vi "Test MQTT-2.2.2-1.vi"(8 "error in (no error)":errorcluster) -> (0 "error out":errorcluster)   [LabVIEW 2013]
uses:
  <vilib>/LabVIEW Open Source Project/MQTT Control Packets/Control Packets/CONNECT/ConnectFlags -- cluster.ctl
  <vilib>/LabVIEW Open Source Project/MQTT Control Packets/Control Packets/SUBACK/Subscription Success Code.ctl
  <vilib>/LabVIEW Open Source Project/MQTT Control Packets/Control Packets/ControlPacket/QualityOfService -- enum.ctl
  <vilib>/LabVIEW Open Source Project/MQTT Control Packets/Control Packets/SUBSCRIBE/Topic Subscription -- cluster.ctl
  <vilib>/LabVIEW Open Source Project/MQTT Control Packets/Control Packets/ControlPacket/ControlPacket.lvclass/ControlPacket.ctl
  <vilib>/addons/_JKI Toolkits/Caraya/classes/Assert/Assert True.vi
  <vilib>/addons/_JKI Toolkits/Caraya/classes/Test/Test.lvclass
  <vilib>/LabVIEW Open Source Project/MQTT Control Packets/Control Packets/ControlPacket/ControlPacket.lvclass
  <vilib>/addons/_JKI Toolkits/Caraya/classes/Assert/Assert.lvclass
  <vilib>/LabVIEW Open Source Project/MQTT Control Packets/Control Packets/CONNECT/CONNECT.lvclass
  <vilib>/LabVIEW Open Source Project/MQTT Control Packets/Control Packets/CONNACK/CONNACK.lvclass
  <vilib>/LabVIEW Open Source Project/MQTT Control Packets/Control Packets/DISCONNECT/DISCONNECT.lvclass
  <vilib>/LabVIEW Open Source Project/MQTT Control Packets/Control Packets/PINGREQ/PINGREQ.lvclass
  <vilib>/LabVIEW Open Source Project/MQTT Control Packets/Control Packets/PINGRESP/PINGRESP.lvclass
  <vilib>/LabVIEW Open Source Project/MQTT Control Packets/Control Packets/PUBACK/PUBACK.lvclass
  <vilib>/LabVIEW Open Source Project/MQTT Control Packets/Control Packets/PUBCOMP/PUBCOMP.lvclass
  <vilib>/LabVIEW Open Source Project/MQTT Control Packets/Control Packets/UNSUBSCRIBE/UNSUBSCRIBE.lvclass
  <vilib>/LabVIEW Open Source Project/MQTT Control Packets/Control Packets/UNSUBACK/UNSUBACK.lvclass
  <vilib>/LabVIEW Open Source Project/MQTT Control Packets/Control Packets/SUBSCRIBE/SUBSCRIBE.lvclass
  <vilib>/LabVIEW Open Source Project/MQTT Control Packets/Control Packets/SUBACK/SUBACK.lvclass
  <vilib>/LabVIEW Open Source Project/MQTT Control Packets/Control Packets/PUBREL/PUBREL.lvclass
  <vilib>/LabVIEW Open Source Project/MQTT Control Packets/Control Packets/PUBREC/PUBREC.lvclass
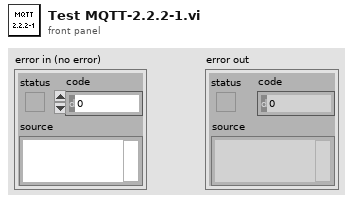
[diagram p1: front panel]
types:
  T1 = typedef "MQTT_Control_Packets.lvlib/SUBSCRIBE.lvclass/Topic Subscription -- cluster.ctl" = cluster{"Topic Filter":string, "QoS":T2}
  T2 = typedef "MQTT_Control_Packets.lvlib/ControlPacket.lvclass/QualityOfService -- enum.ctl" = enum16{"0 (At Most Once)", "1 (At Least Once)", "2 (Exactly Once)"}
  T3 = typedef "MQTT_Control_Packets.lvlib/SUBACK.lvclass/Subscription Success Code.ctl" = cluster{"Subscription Failure":bool, "QoS":T2}
  T4 = typedef "MQTT_Control_Packets.lvlib/CONNECT.lvclass/ConnectFlags -- cluster.ctl" = cluster{"Reserved":bool, "Clean Session":bool, "Will Flag":bool, "Will QoS 1":bool, "Will QoS 2":bool, "Will Retain":bool, "Password Flag":bool, "User Name Flag":bool}
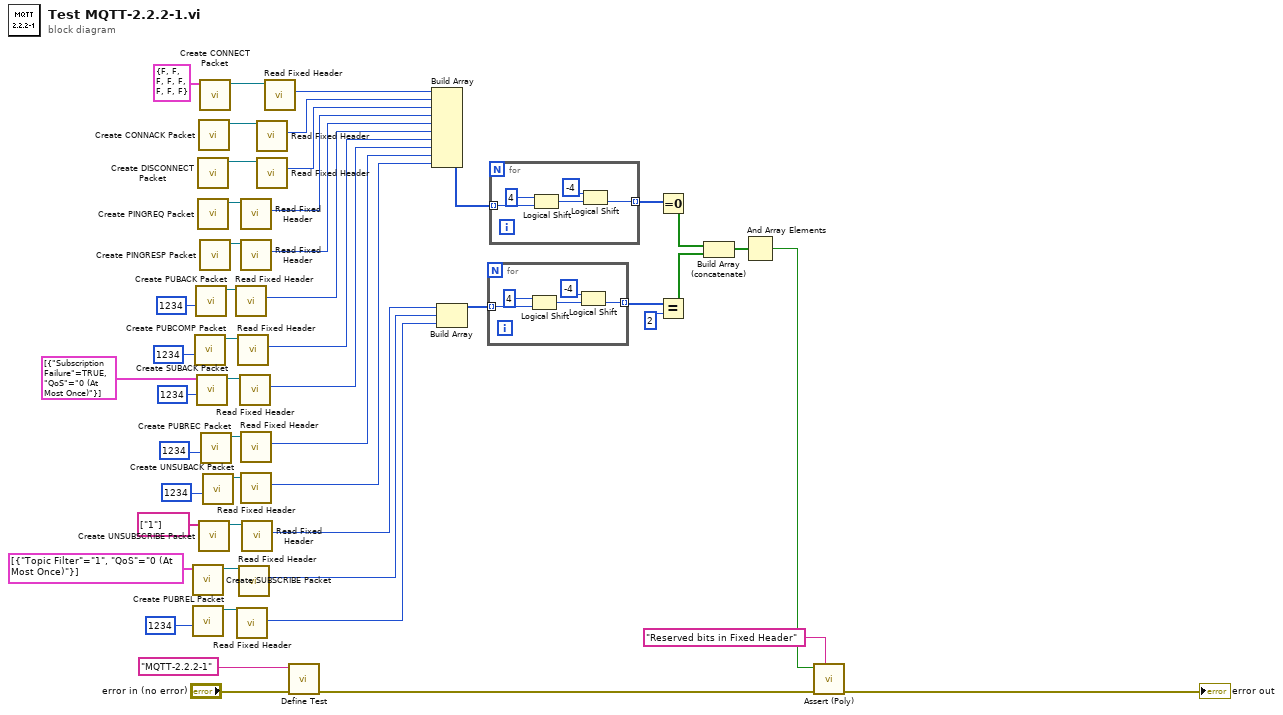
[diagram p0: block diagram]
diagram:
  n1 = call <vilib>:"Create SUBSCRIBE Packet.vi"("Topic Subscriptions"=T1[] [{"Topic Filter"="1", "QoS"=enum."0 (At Most Once)"}]) -> ("SUBSCRIBE out"=w24:refnum<class "SUBSCRIBE.lvclass">)  [unwired: 9 in, 1 out]
  n2 = call <vilib>:"Create PUBREL Packet.vi"("Packet ID"=u16 1234) -> ("PUBREL out"=w31:refnum<class "PUBREL.lvclass">)  [unwired: 9 in, 1 out]
  n3 = call <vilib>:"Create PUBCOMP Packet.vi"("Packet ID"=u16 1234) -> ("PUBCOMP out"=w37:refnum<class "PUBCOMP.lvclass">)  [unwired: 9 in, 1 out]
  n4 = call <vilib>:"Create PUBACK Packet.vi"("Packet ID"=u16 1234) -> ("PUBACK out"=w39:refnum<class "PUBACK.lvclass">)  [unwired: 9 in, 1 out]
  n5 = call <vilib>:"Create SUBACK Packet.vi"("Packet ID"=u16 1234, "Return Codes"=T3[] [{"Subscription Failure"=TRUE, "QoS"=enum."0 (At Most Once)"}]) -> ("SUBACK"=w33:refnum<class "SUBACK.lvclass">)  [unwired: 8 in, 1 out]
  n6 = call <vilib>:"Create DISCONNECT Packet.vi"() -> ("DISCONNECT"=w43:refnum<class "DISCONNECT.lvclass">)  [unwired: 10 in, 1 out]
  n7 = call <vilib>:"Create PINGREQ Packet.vi"() -> ("PINGREQ out"=w42:refnum<class "PINGREQ.lvclass">)  [unwired: 10 in, 1 out]
  n8 = call <vilib>:"Create CONNACK Packet.vi"() -> ("CONNACK"=w44:refnum<class "CONNACK.lvclass">)  [unwired: 10 in, 1 out]
  n9 = call <vilib>:"Create UNSUBSCRIBE Packet.vi"("Topic Subscriptions"=string[] ["1"]) -> ("UNSUBSCRIBE out"=w36:refnum<class "UNSUBSCRIBE.lvclass">)  [unwired: 9 in, 1 out]
  n10 = call <vilib>:"Create CONNECT Packet.vi"("Connect Flags"=T4 {"Reserved"=FALSE, "Clean Session"=FALSE, "Will Flag"=FALSE, "Will QoS 1"=FALSE, "Will QoS 2"=FALSE, "Will Retain"=FALSE, "Password Flag"=FALSE, "User Name Flag"=FALSE}) -> ("CONNECT"=w45:refnum<class "CONNECT.lvclass">)  [unwired: 9 in, 1 out]
  n11 = call <vilib>:"Create PINGRESP Packet.vi"() -> ("PINGRESP out"=w41:refnum<class "PINGRESP.lvclass">)  [unwired: 10 in, 1 out]
  n12 = call <vilib>:"Create PUBREC Packet.vi"("Packet ID"=u16 1234) -> ("PUBREC out"=w29:refnum<class "PUBREC.lvclass">)  [unwired: 9 in, 1 out]
  n13 = call <vilib>:"Create UNSUBACK Packet.vi"("Packet ID"=u16 1234) -> ("UNSUBACK out"=w27:refnum<class "UNSUBACK.lvclass">)  [unwired: 9 in, 1 out]
  n14 = call <vilib>:"Read Fixed Header.vi"("ControlPacket in"=w39) -> ("Fixed Header"=w18:u8)  [unwired: 9 in, 1 out]
  n15 = call <vilib>:"Read Fixed Header.vi"("ControlPacket in"=w31) -> ("Fixed Header"=w10:u8)  [unwired: 9 in, 1 out]
  n16 = call <vilib>:"Read Fixed Header.vi"("ControlPacket in"=w37) -> ("Fixed Header"=w17:u8)  [unwired: 9 in, 1 out]
  n17 = call <vilib>:"Read Fixed Header.vi"("ControlPacket in"=w24) -> ("Fixed Header"=w11:u8)  [unwired: 9 in, 1 out]
  n18 = call <vilib>:"Read Fixed Header.vi"("ControlPacket in"=w33) -> ("Fixed Header"=w14:u8)  [unwired: 9 in, 1 out]
  n19 = call <vilib>:"Read Fixed Header.vi"("ControlPacket in"=w42) -> ("Fixed Header"=w20:u8)  [unwired: 9 in, 1 out]
  n20 = call <vilib>:"Read Fixed Header.vi"("ControlPacket in"=w41) -> ("Fixed Header"=w19:u8)  [unwired: 9 in, 1 out]
  n21 = call <vilib>:"Read Fixed Header.vi"("ControlPacket in"=w29) -> ("Fixed Header"=w16:u8)  [unwired: 9 in, 1 out]
  n22 = call <vilib>:"Read Fixed Header.vi"("ControlPacket in"=w27) -> ("Fixed Header"=w15:u8)  [unwired: 9 in, 1 out]
  n23 = call <vilib>:"Read Fixed Header.vi"("ControlPacket in"=w36) -> ("Fixed Header"=w12:u8)  [unwired: 9 in, 1 out]
  n24 = call <vilib>:"Read Fixed Header.vi"("ControlPacket in"=w44) -> ("Fixed Header"=w22:u8)  [unwired: 9 in, 1 out]
  n25 = call <vilib>:"Read Fixed Header.vi"("ControlPacket in"=w43) -> ("Fixed Header"=w21:u8)  [unwired: 9 in, 1 out]
  n26 = call <vilib>:"Read Fixed Header.vi"("ControlPacket in"=w45) -> ("Fixed Header"=w23:u8)  [unwired: 9 in, 1 out]
  n27 = call <vilib>:"Define Test.vi"("error in (no error)"="error in (no error)", "Label (VI Title)"="MQTT-2.2.2-1") -> ("error out"=w48:errorcluster)  [unwired: 9 in]
  n28 = Build Array(w23, w22, w21, w20, w19, w18, w17, w14, w16, w15) -> (w1:u8[])
  n29 = Build Array(w12, w11, w10) -> (w13:u8[])
  n30 = for {
    tunnel: w13 -> [w55] mode=indexing
    tunnel: [w51] -> w3 mode=indexing
    n31 = Logical Shift(y=i16 4, x=w55) -> (x << y=w53:u8)
    n32 = Logical Shift(y=i16 -4, x=w53) -> (x << y=w51:u8)
  }
  n33 = for {
    tunnel: w1 -> [w60] mode=indexing
    tunnel: [w56] -> w2 mode=indexing
    n34 = Logical Shift(y=i16 4, x=w60) -> (x << y=w58:u8)
    n35 = Logical Shift(y=i16 -4, x=w58) -> (x << y=w56:u8)
  }
  n36 = Equal To 0?(x=w2) -> (x = 0?=w8:bool[])
  n37 = Equal?(x=w3, y=2) -> (x = y?=w7:bool[])
  n38 = Build Array (concatenate)(w8, w7) -> (w6:bool[])
  n39 = And Array Elements(Boolean array=w6) -> (logical AND=w5:bool)
  n40 = call-poly <vilib>:"Assert (Poly).vi"("Label"="Reserved bits in Fixed Header", "error in (no error)"=w48, "True?"=w5) -> ("error out"=→"error out":errorcluster)  [unwired: 8 in]
